vi "Write Field name.vi"(8 "error in (no error)":errorcluster, 10 "Field name":string, 11 "Write FP Control Msg in":refnum<class "Write FP Control Msg.lvclass">) -> (0 "error out":errorcluster, 3 "Write FP Control Msg out":refnum<class "Write FP Control Msg.lvclass">)   [LabVIEW 2016, in "Write FP Control Msg.lvclass"]
uses:
  Write FP Control Msg.lvclass
  Write FP Control Msg.lvclass/Write FP Control Msg.ctl
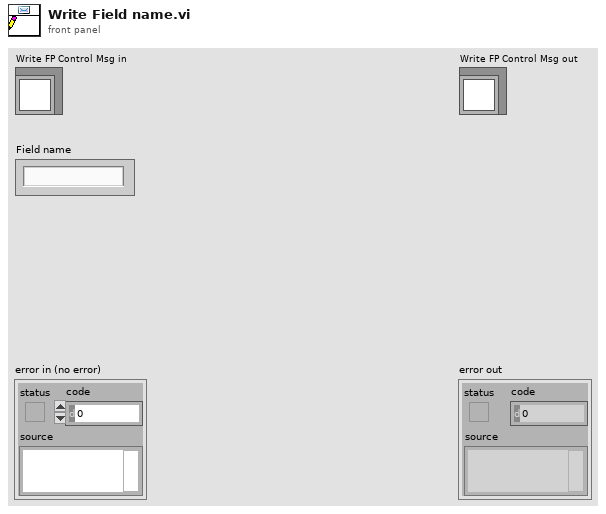
[diagram p1: front panel]
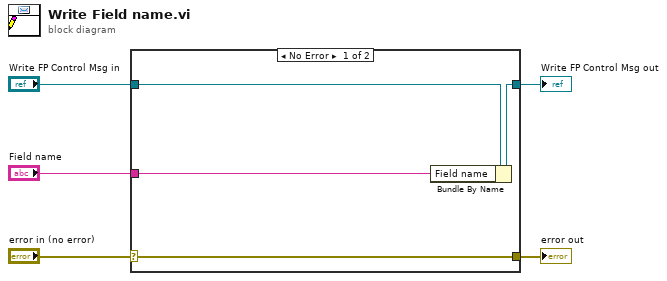
[diagram p0: block diagram]
diagram:
  n1 = case shown="No Error" "error in (no error)" {
    selector: "error in (no error)" -> [w9 w10]
    tunnel: [w9 w10] -> w4
    tunnel: [w7 w11] -> w2
    tunnel: "Write FP Control Msg in" -> [w8 w11]
    tunnel: "Field name" -> [w6 _]
    frame No Error {
      n2 = Bundle By Name(cluster=w8, "Field name"=w6) -> (w7:refnum<class "Write FP Control Msg.lvclass">)
    }
    frame Error {
    }
  }
  "error out" <- w4
  "Write FP Control Msg out" <- w2
